vi "Main.vi"() -> ()   [LabVIEW 2017]
uses:
  TypeDefs/Listbox.ctl
  TypeDefs/Multicolumn.ctl
  TypeDefs/TabControl.ctl
  TypeDefs/Transparent String.ctl
  TypeDefs/DCP and LLDP Cluster.ctl
  TypeDefs/DCP ARRAY.ctl
  TypeDefs/Profinet Ident.ctl
  TypeDefs/LLDP ARRAY.ctl
  TypeDefs/LLDP.ctl
  Lib/WinPcap/lvwpcap.lvlib
panel:
  out "Program State":T1
  in  "Configuration Tab":bool
  in  "Scan Tab":bool
  in  "List of accessible devices:":T2
  in  "Tab Control":T3
  in  "Cancel Scan":bool
  in  "Network Adapters":T4
  in  "Scan Button":bool
  in  "Input parameter 3":string
  in  "Input parameter 2":string
  in  "Cancel Set":bool
  in  "Flash LED":bool
  in  "Set Button":bool
  in  "Input parameter 1":string
  in  "Choose Mode":T4
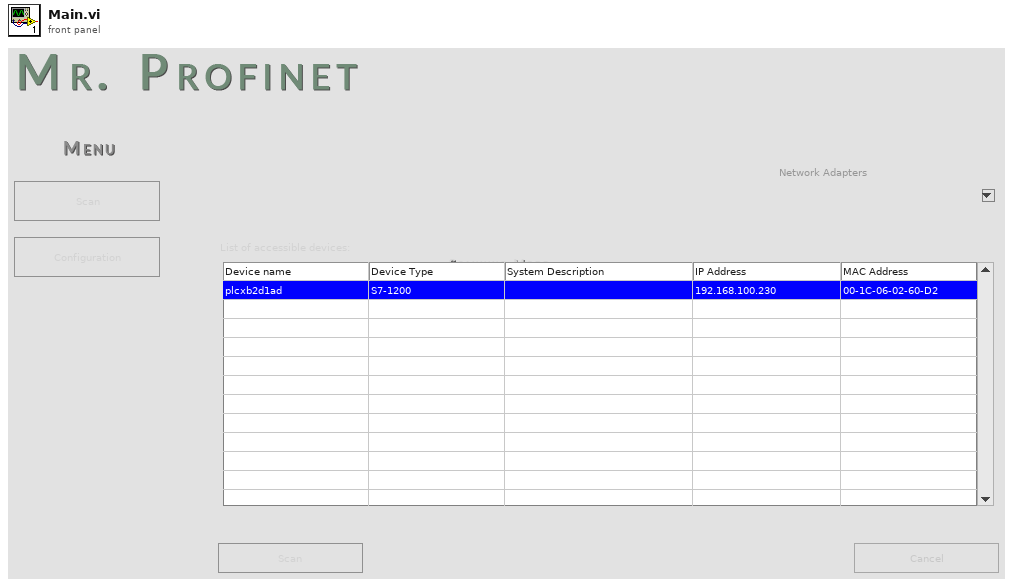
[diagram p1: front panel]
types:
  T1 = typedef "Transparent String.ctl" = string
  T2 = typedef "Multicolumn.ctl" = i32
  T3 = typedef "TabControl.ctl" = enum32{"Scan", "Configuration"}
  T4 = typedef "Listbox.ctl" = string
  T5 = enum32{"invalid app kind", "Development System", "Run Time System", "Student Edition", "Embedded LabVIEW", "Evaluation", "Custom"}
  T6 = enum8{"Enabled", "Disabled", "Disabled and Grayed Out"}
  T7 = enum32{"Invalid", "Standard", "Closed", "Hidden", "Minimized", "Maximized"}
  T8 = typedef "DCP and LLDP Cluster.ctl" = cluster{"DCP":T9, "LLDP":T11}
  T9 = typedef "DCP ARRAY.ctl" = T10[]
  T10 = typedef "Profinet Ident.ctl" = cluster{"Device Vendor Value":string, "Name Of Station":string, "IP Address":string, "Subnet Mask":string, "Default Gateway":string, "MAC Address":string, "MAC Address HEX":string, "System Description ":string}
  T11 = typedef "LLDP ARRAY.ctl" = T12[]
  T12 = typedef "LLDP.ctl" = cluster{"Chasis Subtype":string, "Port Subtype":string, "Port Description":string, "System Name":string, "System Description":string, "IP Address":string, "MAC Address":string, "MAC Address HEX":string}
  T13 = cluster{"Core":cluster{"Current VI Reference":refnum<vi>, "Close Panel on Exit?":bool}, "Scanner Data":T8, "Accesible Devices":string[][], "Interfaces":string[], "Interface index":i32, "Pcap Reference":u32, "Send parameters":cluster{"MAC Address":string, "Mode":string, "Parameter 1":string, "Parameter 2":string, "Parameter 3":string}}
  T14 = cluster{"MAC Address":string, "Mode":string, "Parameter 1":string, "Parameter 2":string, "Parameter 3":string}
  T15 = cluster{"Current VI Reference":refnum<vi>, "Close Panel on Exit?":bool}
  T16 = typedef "Control majster 5.ctl" = string
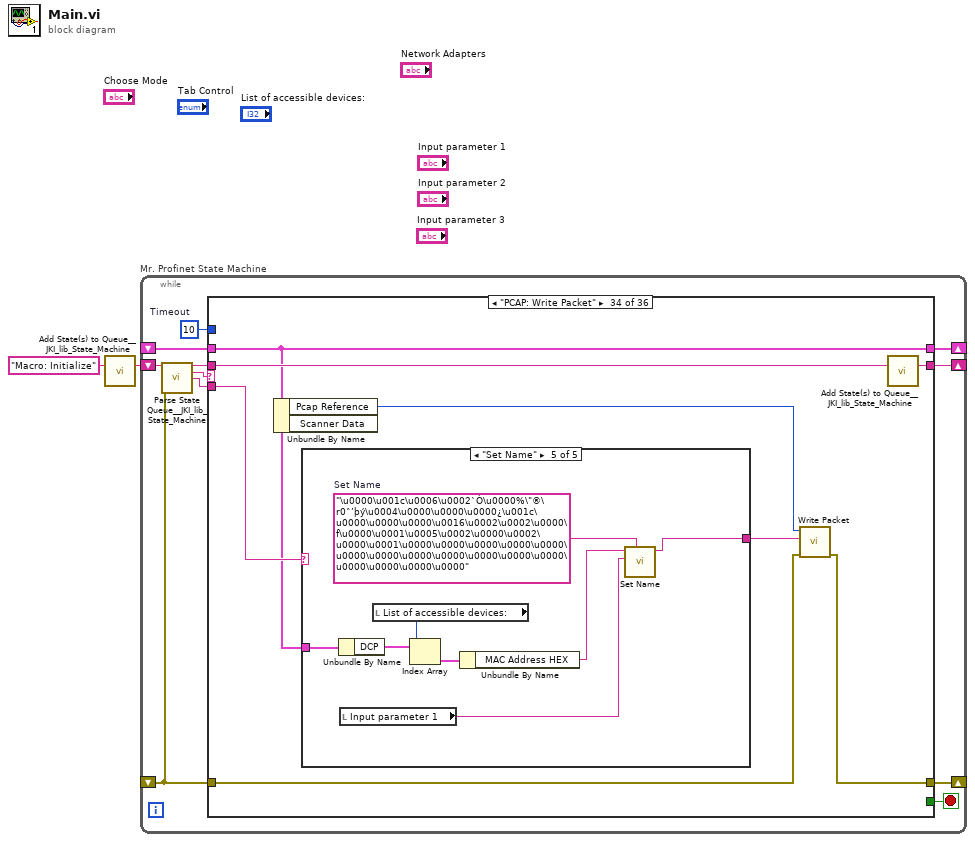
[diagram p0: block diagram]
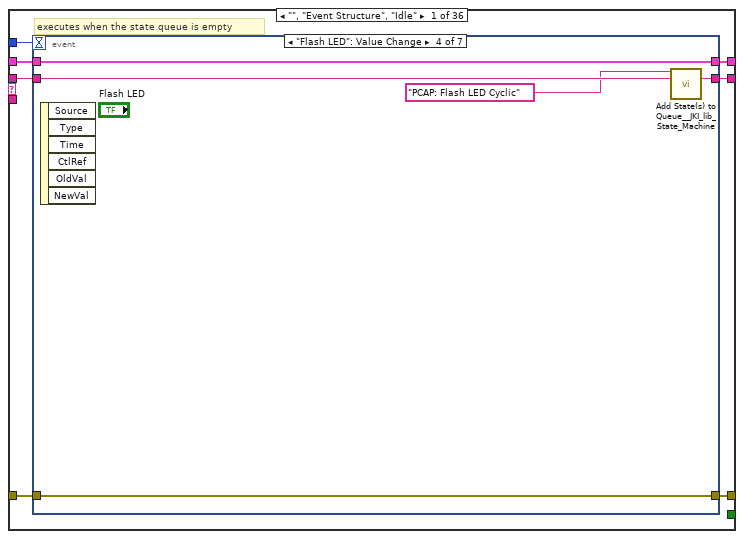
[diagram p2: hidden frame]
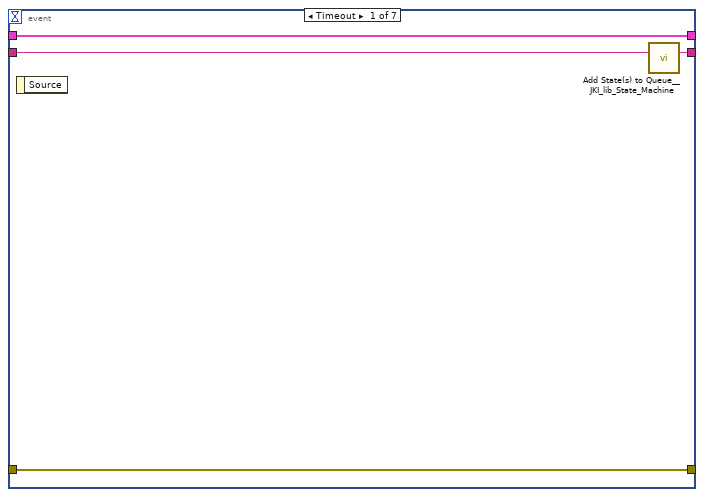
[diagram p3: hidden frame]
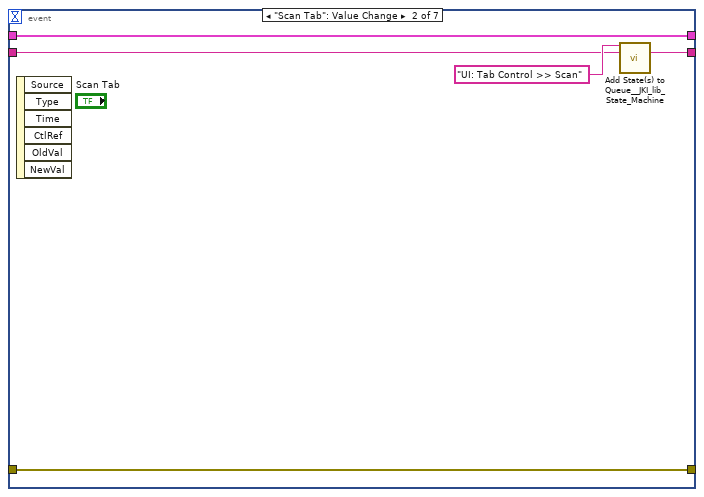
[diagram p4: hidden frame]
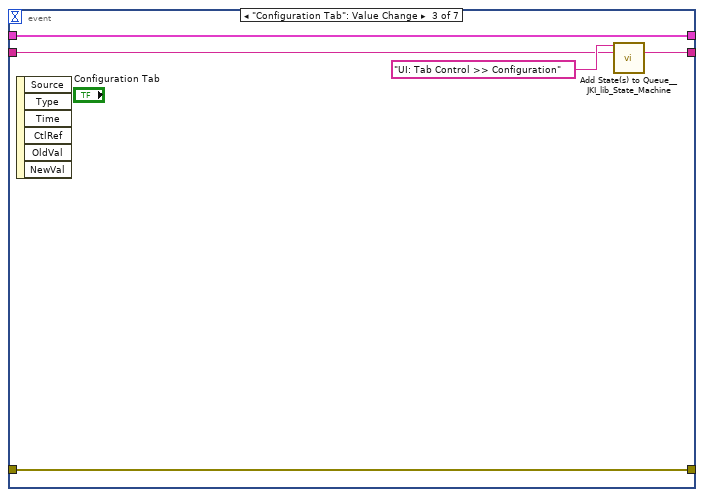
[diagram p5: hidden frame]
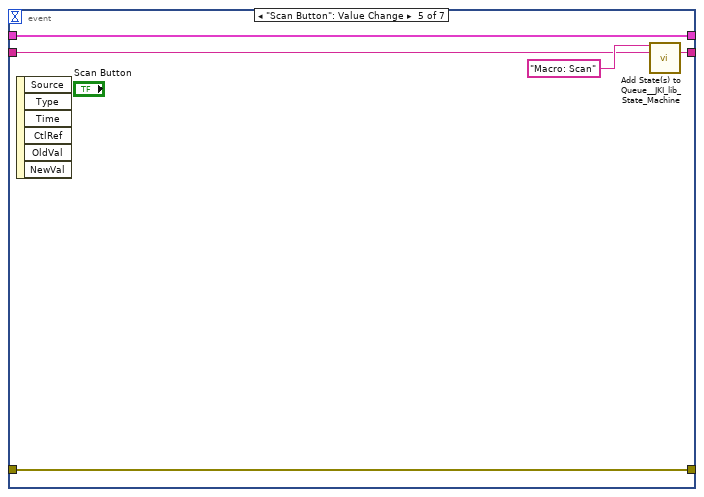
[diagram p6: hidden frame]
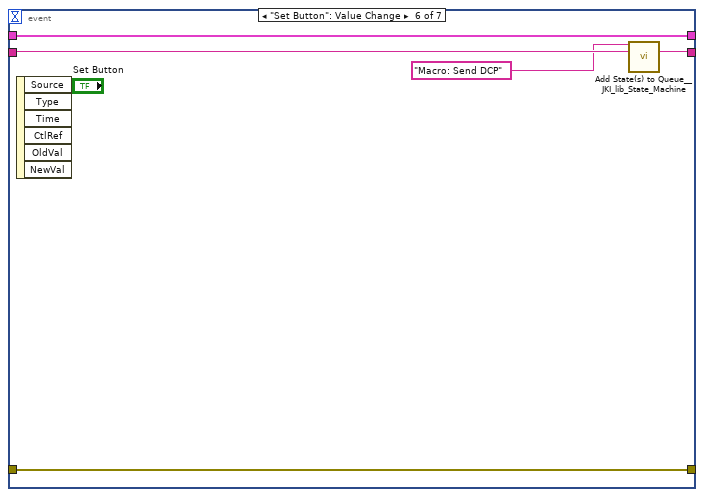
[diagram p7: hidden frame]
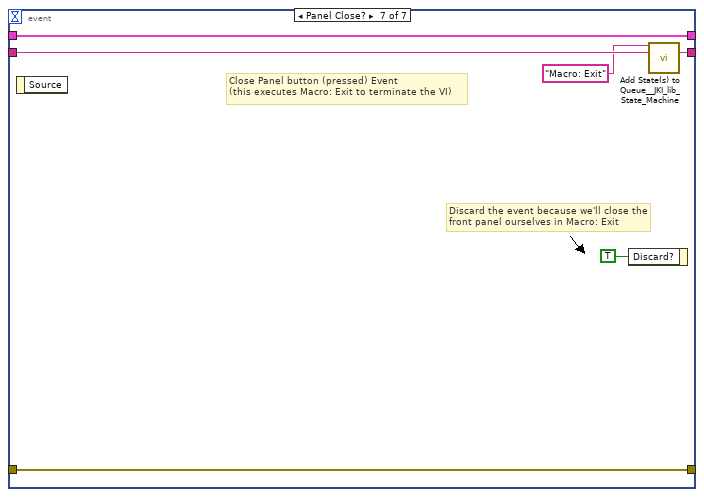
[diagram p8: hidden frame]
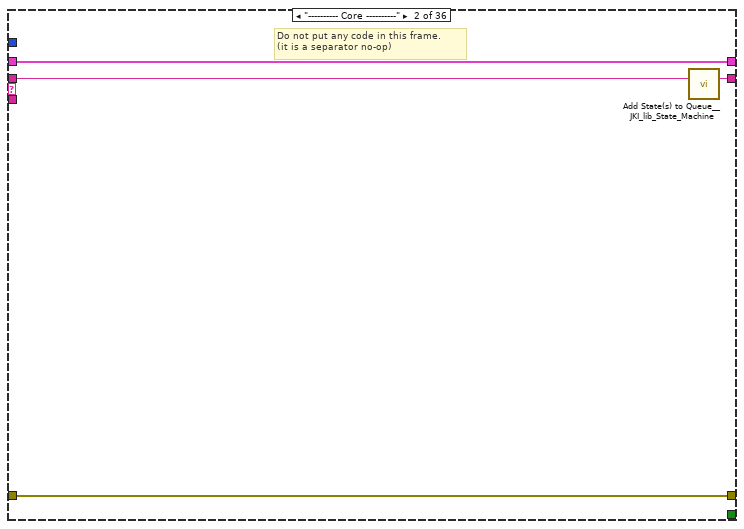
[diagram p9: hidden frame]
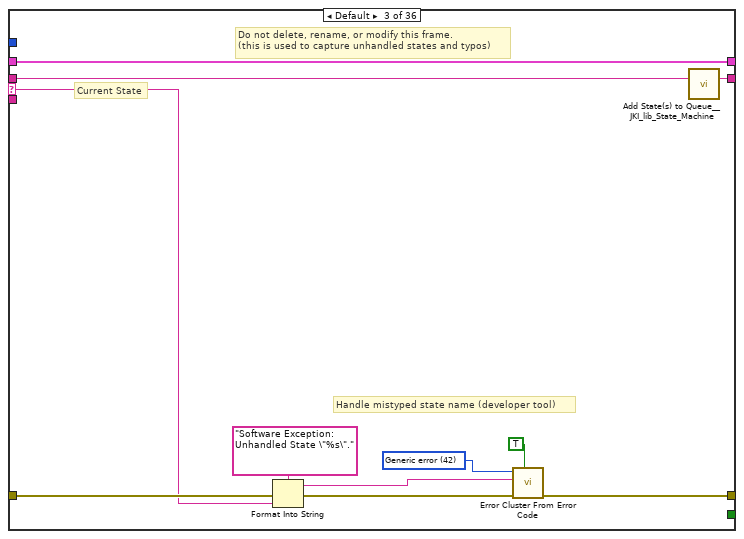
[diagram p10: hidden frame]
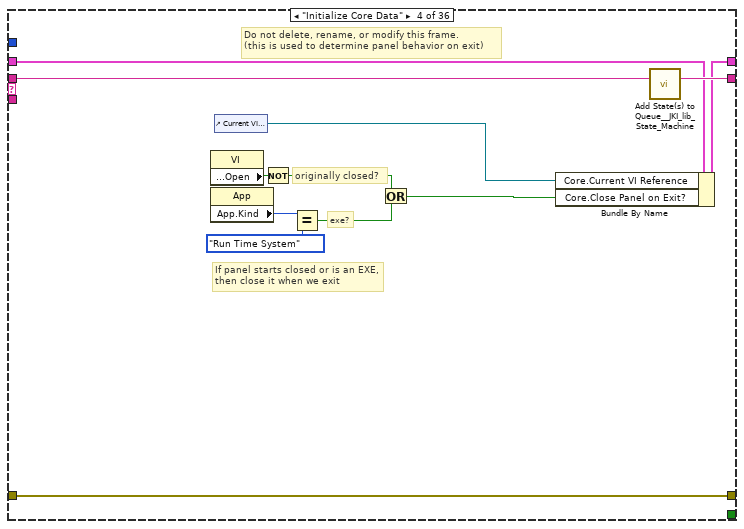
[diagram p11: hidden frame]
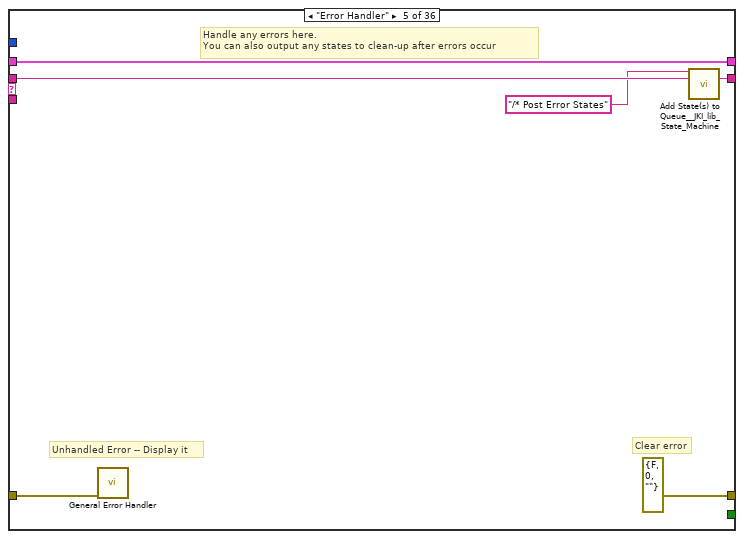
[diagram p12: hidden frame]
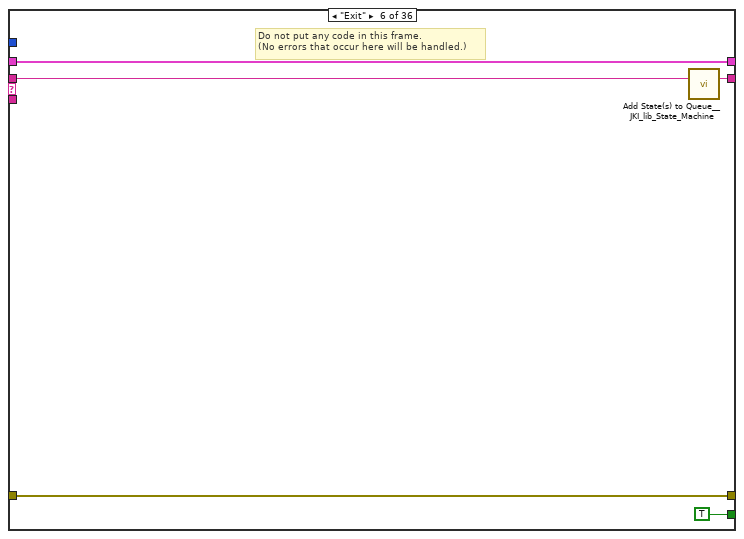
[diagram p13: hidden frame]
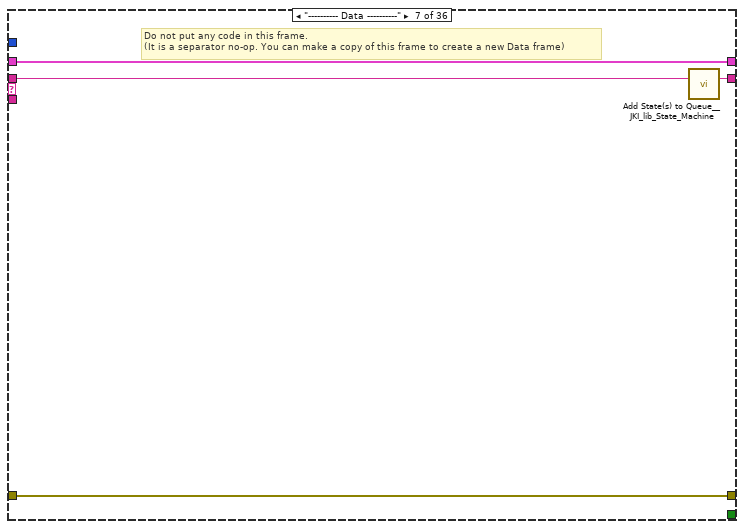
[diagram p14: hidden frame]
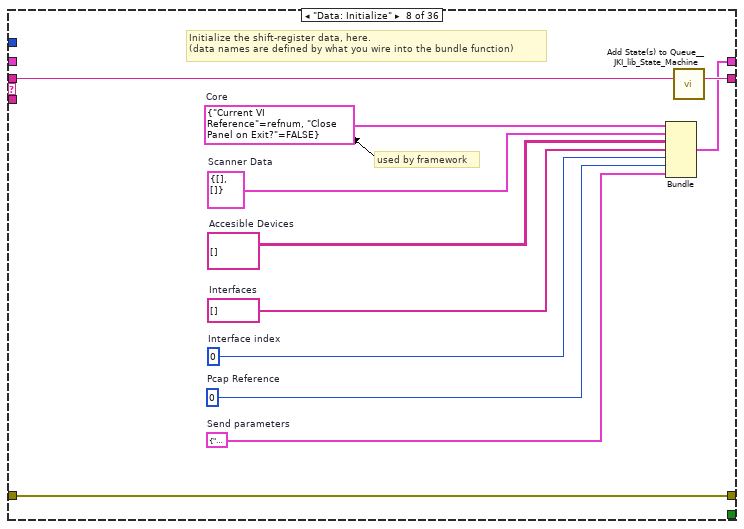
[diagram p15: hidden frame]
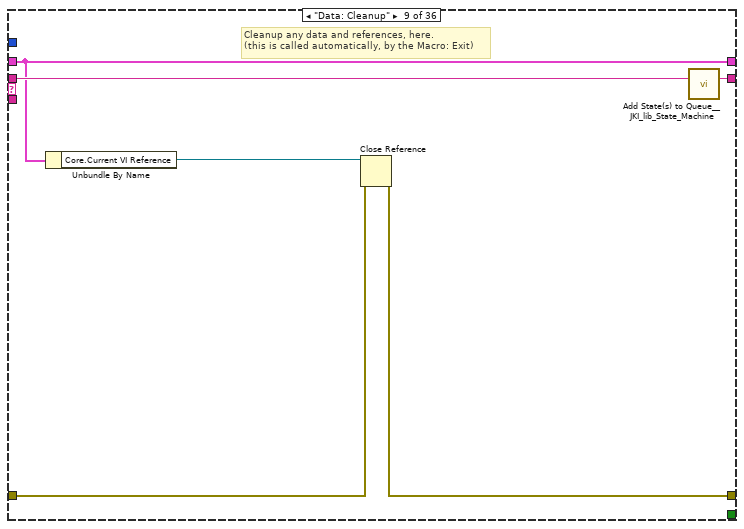
[diagram p16: hidden frame]
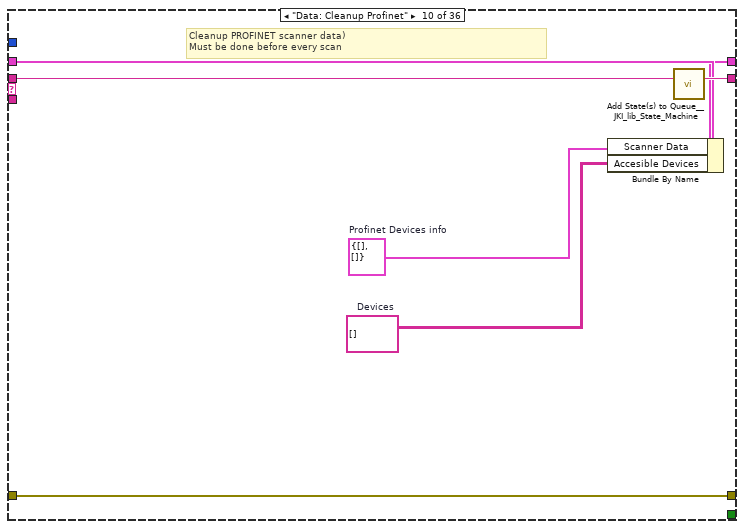
[diagram p17: hidden frame]
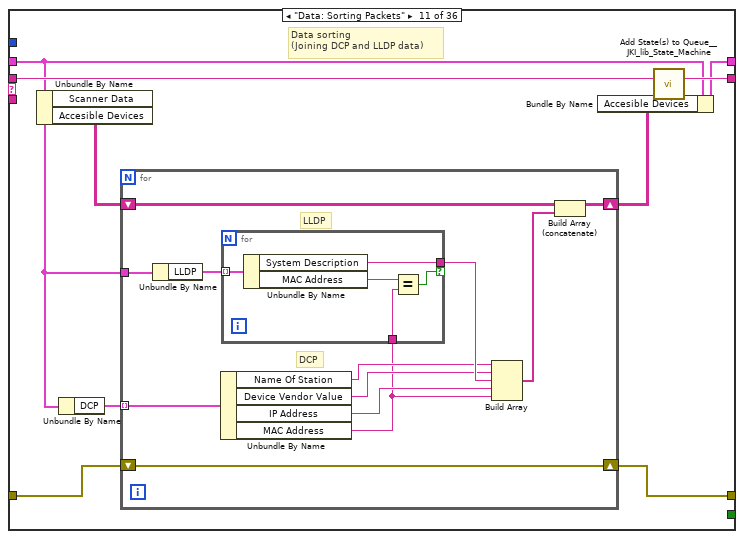
[diagram p18: hidden frame]
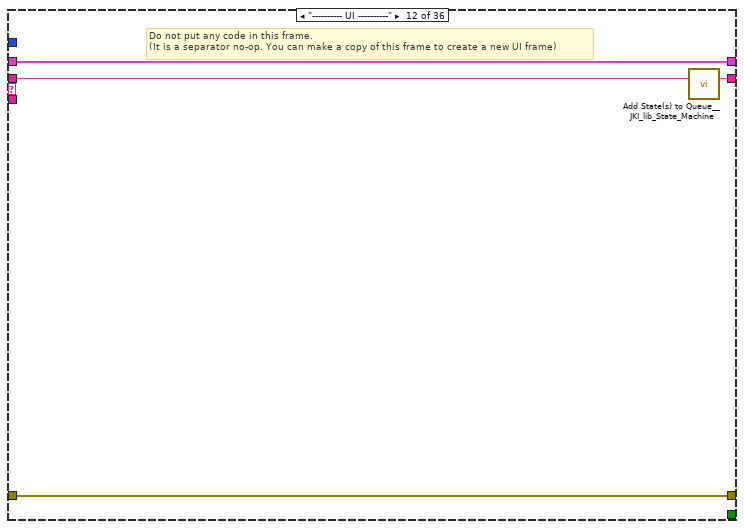
[diagram p19: hidden frame]
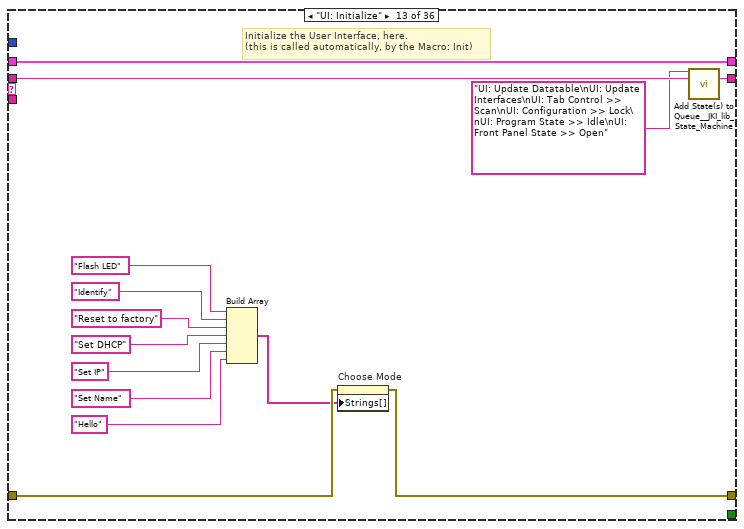
[diagram p20: hidden frame]
diagram:
  n1 = call <vilib>:"Add State(s) to Queue__JKI_lib_State_Machine.vi"("State(s) in (\"\")"="Macro: Initialize") -> ("States Out"=w2:string)  [unwired: 14 in]
  n2 = while "Mr. Profinet State Machine" {
    shift-right: [w6] -> _
    shift-left: _ -> [w5]
    shift-right: [w9] -> _
    shift-left: _ -> [w3]
    shift-right: [w8] -> _
    shift-left: w2 -> [w10]
    stop <- w7 stop-if-true
    w4 = 10  # Timeout
    n3 = call <vilib>:"Parse State Queue__JKI_lib_State_Machine.vi"("State Queue"=w10, "Error In (no error)"=w3) -> ("Remaining States"=w12:string, "Current State"=w13:string, "Arguments"=w11:string)  [unwired: 11 in]
    n4 = case shown="\"PCAP: Write Packet\"" w13 {
      selector: w13 -> [_ _ w60 _ _ _ _ _ _ _ _ _ _ _ _ _ _ _ _ _ _ _ _ _ _ _ _ _ _ _ _ _ _ _ _ _]
      tunnel: w12 -> [w20 w59 w64 w82 w88 w93 w97 w108 w114 w121 w131 w152 w166 w172 w178 w184 w194 w212 w230 w242 w252 w263 w289 w294 w299 w304 w312 w317 w327 w331 w345 w359 w366 w379 w425 w443]
      tunnel: w11 -> [_ _ _ _ _ _ _ _ _ _ _ _ _ _ _ w179 w189 w207 w225 w237 w247 w257 _ _ _ _ _ _ _ _ _ _ _ w373 _ _]
      tunnel: w5 -> [w18 w56 w62 w73 w85 w91 w94 _ w109 w118 w128 w149 w164 w170 w173 w182 w192 w210 w228 w240 w250 w259 w286 w291 w296 w301 w310 w314 w324 w328 w334 w352 w364 w377 w421 w438]
      tunnel: [w17 w57 w66 w79 errorcluster {"status"=FALSE, "code"=0, "source"=""} ("error out") w90 w95 w105 w110 w119 w126 w150 w161 w167 w174 w180 w190 w208 w226 w238 w248 w260 w287 w292 w297 w302 w308 w315 w325 w329 w336 w355 w362 w376 w418 w439] -> w9
      tunnel: w3 -> [w16 w57 w65 w79 w84 w90 w95 w105 w111 w119 w129 w150 w162 w168 w175 w181 w191 w209 w227 w239 w249 w261 w287 w292 w297 w302 w309 w315 w325 w329 w343 w356 w363 w375 w423 w441]
      tunnel: [w19 w58 w63 w81 w87 w92 w96 w107 w113 w120 w130 w151 w165 w171 w177 w183 w193 w211 w229 w241 w251 w262 w288 w293 w298 w303 w311 w316 w326 w330 w344 w358 w365 w378 w424 w442] -> w8
      tunnel: [_ _ _ _ _ TRUE _ _ _ _ _ _ _ _ _ _ _ _ _ _ _ _ _ _ _ _ _ _ _ _ _ _ _ _ _ _] -> w7
      tunnel: [w15 w56 w62 w80 w85 w91 w94 w106 w109 w116 w127 w149 w164 w170 w173 w182 w192 w210 w228 w240 w250 w259 w286 w291 w296 w301 w310 w314 w324 w328 w333 w351 w364 w377 w420 w438] -> w6
      tunnel: w4 -> [w14 _ _ _ _ _ _ _ _ _ _ _ _ _ _ _ _ _ _ _ _ _ _ _ _ _ _ _ _ _ _ _ _ _ _ _]
      frame "", "Event Structure", "Idle" {
        # "executes when the state queue is empty"
        n5 = event shown="[3] \"Flash LED\": Value Change" {
          selector: _ -> [_ _ _ _ _ _ _]
          dyn-events: _ -> [_ _ _ _ _ _ _]
          timeout: w14 -> [_ _ _ _ _ _ _]
          tunnel: w20 -> [w24 w25 w31 w37 w42 w47 w55]
          tunnel: [w23 w26 w32 w38 w43 w48 w54] -> w19
          tunnel: w18 -> [w21 w29 w34 w39 w41 w49 w52]
          tunnel: [w22 w28 w30 w36 w40 w45 w53] -> w17
          tunnel: w16 -> [w22 w28 w30 w36 w40 w45 w53]
          tunnel: [w21 w29 w34 w39 w41 w49 w52] -> w15
          event Timeout {
            n6 = event-data() -> ()  [unwired: 1 in, 1 out]
            n7 = call <vilib>:"Add State(s) to Queue__JKI_lib_State_Machine.vi"("State(s) in (\"\")"=w24) -> ("States Out"=w23:string)  [unwired: 14 in]
          }
          event "Scan Tab": Value Change {
            n8 = event-data() -> ()  [unwired: 1 in, 6 out]
            n9 = call <vilib>:"Add State(s) to Queue__JKI_lib_State_Machine.vi"("State(s) in Front (\"\")"="UI: Tab Control >> Scan", "State(s) in (\"\")"=w25) -> ("States Out"=w26:string)  [unwired: 13 in]
          }
          event "Configuration Tab": Value Change {
            n10 = event-data() -> ()  [unwired: 1 in, 6 out]
            n11 = call <vilib>:"Add State(s) to Queue__JKI_lib_State_Machine.vi"("State(s) in Front (\"\")"="UI: Tab Control >> Configuration", "State(s) in (\"\")"=w31) -> ("States Out"=w32:string)  [unwired: 13 in]
          }
          event "Flash LED": Value Change {
            n12 = event-data() -> ()  [unwired: 1 in, 6 out]
            n13 = call <vilib>:"Add State(s) to Queue__JKI_lib_State_Machine.vi"("State(s) in Front (\"\")"="PCAP: Flash LED Cyclic" ("State(s) in Front (\"\")"), "State(s) in (\"\")"=w37) -> ("States Out"=w38:string)  [unwired: 13 in]
          }
          event "Scan Button": Value Change {
            n14 = event-data() -> ()  [unwired: 1 in, 6 out]
            n15 = call <vilib>:"Add State(s) to Queue__JKI_lib_State_Machine.vi"("State(s) in Front (\"\")"="Macro: Scan", "State(s) in (\"\")"=w42) -> ("States Out"=w43:string)  [unwired: 13 in]
          }
          event "Set Button": Value Change {
            n16 = event-data() -> ()  [unwired: 1 in, 6 out]
            n17 = call <vilib>:"Add State(s) to Queue__JKI_lib_State_Machine.vi"("State(s) in Front (\"\")"="Macro: Send DCP", "State(s) in (\"\")"=w47) -> ("States Out"=w48:string)  [unwired: 13 in]
          }
          event Panel Close? {
            # "Discard the event because we'll close the front panel ourselves in Macro: Exit"
            # "Close Panel button (pressed) Event\n(this executes Macro: Exit to terminate the VI)"
            n18 = event-data() -> ()  [unwired: 1 in, 1 out]
            n19 = event-data("Discard?"=TRUE) -> ()  [unwired: 1 in, 1 out]
            n20 = call <vilib>:"Add State(s) to Queue__JKI_lib_State_Machine.vi"("State(s) in Front (\"\")"="Macro: Exit", "State(s) in (\"\")"=w55) -> ("States Out"=w54:string)  [unwired: 13 in]
          }
        }
      }
      frame "---------- Core ----------" {
        # "Do not put any code in this frame.\n(it is a separator no-op)"
        n21 = call <vilib>:"Add State(s) to Queue__JKI_lib_State_Machine.vi"("State(s) in (\"\")"=w59) -> ("States Out"=w58:string)  [unwired: 14 in]
      }
      frame Default {
        w69 = 42 items=["No error", "Argument error", "Memory is full", "Out of zone", "End of file", "File already open", "Generic file I/O error", "File not found", "File permission error", "Disk is full", "Duplicate path", "Too many files open", "System feature not enabled", "Resource file not found", "Cannot add resource", "Resource not found", "Image not found", "Image memory error", "Pen does not exist", "Config type invalid", "Config token not found", "Config parse error", "Config memory error", "Bad external code format", "Bad external code offset", "External code not present", "Null window", "Destroy window error", "Null menu", "Print aborted", "Bad print record", "Print driver error", "Windows error during printing", "Memory error during printing", "Print dialog error", "Generic print error", "Invalid device refnum", "Device not found", "Device parameter error", "Device unit error", "Cannot open device", "Device call aborted", "Generic error", "Cancelled by user", "Object ID too low", "Object ID too high", "Object not in heap", "Unknown heap", "Unknown object (invalid DefProc)", "Unknown object (DefProc not in table)", "Message out of range", "Invalid (null) method", "Unknown message", "Manager call not supported", "Bad address", "Network operation in progress", "Network operation timed out", "Connection is busy", "Network attribute not supported", "Network error", "Address in use", "System out of memory", "Connection aborted", "Connection refused", "Not connected", "Already connected", "Connection closed", "Initialization error (interapplication manager)", "Bad occurrence", "Wait on unbound occurrence handler", "Occurrence queue overflow", "Datalog type conflict", "Unused", "Unrecognized type (interapplication manager)", "Memory corrupt", "Failed to make temporary DLL", "Old CIN version", "Drag socket not found", "Failed to load drop-object", "Failed to register OLE object", "Failed to release OLE object", "Format specifier type mismatch", "Unknown format specifier", "Too few format specifiers", "Too many format specifiers", "Scan failed", "Newer CIN version", "Error converting to variant", "Runtime menu error", "Password tampered", "Variant attribute not found", "Incompatible variant data type", "Event data is not available", "Event Store is not present", "Occurrence is not found", "Event Queue is not created", "Event info is not available", "Refnum passed is NULL", "Error retrieving Class GUID", "Error retrieving CoClass GUID", "Error retrieving TypeLib GUID.", "Bad built application magic bytes.", "Specific driver is different from the specific driver associated with the Logical Name.", "There is no session opened to the class driver.", "Max Error", "MAX - Error with config objects", "MAX - Error loading configuration", "MAX - Group not supported"]
        # "Current State"
        # "Do not delete, rename, or modify this frame.\n(this is used to capture unhandled states and typos)"
        # "Handle mistyped state name (developer tool)"
        n22 = Format Into String(format string="Software Exception: Unhandled State \"%s\"." ("message"), error in=w65, w60) -> (resulting string=w68:string, error out=w67:errorcluster)  [unwired: 1 in]
        n23 = call <vilib>:"Error Cluster From Error Code.vi"("show call chain? (False)"=TRUE, "error in (no error)"=w67, "error message (\"\")"=w68, "error code (0)"=w69) -> ("error out"=w66:errorcluster)  [unwired: 5 in]
        n24 = call <vilib>:"Add State(s) to Queue__JKI_lib_State_Machine.vi"("State(s) in (\"\")"=w64) -> ("States Out"=w63:string)  [unwired: 14 in]
      }
      frame "Initialize Core Data" {
        # "Do not delete, rename, or modify this frame.\n(this is used to determine panel behavior on exit)"
        # "originally closed?"
        # "exe?"
        # "If panel starts closed or is an EXE, then close it when we exit"
        n25 = property class="VI"() -> ("Front Panel.Open"=w78:bool)  [unwired: 2 in, 2 out]
        n26 = property class="App"() -> ("App.Kind"=w77:T5)  [unwired: 2 in, 2 out]
        n27 = control-ref of="Current VI Reference"() -> (w71:refnum<vi>)
        n28 = Not(x=w78) -> (.not. x?=w75:bool)
        n29 = Equal?(x=w77, y=T5."Run Time System" ("Application:Kind")) -> (x = y?=w74:bool)
        n30 = Or(x=w75, y=w74) -> (x .or. y?=w72:bool)
        n31 = Bundle By Name(cluster=w73, "Core.Current VI Reference"=w71, "Core.Close Panel on Exit?"=w72) -> (w80:T13)
        n32 = call <vilib>:"Add State(s) to Queue__JKI_lib_State_Machine.vi"("State(s) in (\"\")"=w82) -> ("States Out"=w81:string)  [unwired: 14 in]
      }
      frame "Error Handler" {
        # "Unhandled Error -- Display it"
        # "Handle any errors here.\nYou can also output any states to clean-up after errors occur"
        # "Clear error"
        n33 = call <vilib>:"General Error Handler.vi"("error in (no error)"=w84) -> ()  [unwired: 10 in, 5 out]
        n34 = call <vilib>:"Add State(s) to Queue__JKI_lib_State_Machine.vi"("State(s) in Front (\"\")"="/* Post Error States", "State(s) in (\"\")"=w88) -> ("States Out"=w87:string)  [unwired: 13 in]
      }
      frame "Exit" {
        # "Do not put any code in this frame.\n(No errors that occur here will be handled.)"
        n35 = call <vilib>:"Add State(s) to Queue__JKI_lib_State_Machine.vi"("State(s) in (\"\")"=w93) -> ("States Out"=w92:string)  [unwired: 14 in]
      }
      frame "---------- Data ----------" {
        # "Do not put any code in this frame.\n(It is a separator no-op. You can make a copy of this frame to create a new Data frame)"
        n36 = call <vilib>:"Add State(s) to Queue__JKI_lib_State_Machine.vi"("State(s) in (\"\")"=w97) -> ("States Out"=w96:string)  [unwired: 14 in]
      }
      frame "Data: Initialize" {
        w98 = T14 {"MAC Address"="", "Mode"="", "Parameter 1"="", "Parameter 2"="", "Parameter 3"=""}  # Send parameters
        w99 = string[][] []  # Accesible Devices
        w104 = T8 {"DCP"=[], "LLDP"=[]}  # Scanner Data
        w102 = u32 0  # Pcap Reference
        w101 = 0  # Interface index
        w100 = string[] []  # Interfaces
        w103 = T15 {"Current VI Reference"=refnum, "Close Panel on Exit?"=FALSE}  # Core
        # "used by framework"
        # "Initialize the shift-register data, here.\n(data names are defined by what you wire into the bundle function)"
        n37 = Bundle("Core"=w103, "Scanner Data"=w104, "Accesible Devices"=w99, "Interfaces"=w100, "Interface index"=w101, "Pcap Reference"=w102, "Send parameters"=w98) -> (w106:T13)  [unwired: 1 in]
        n38 = call <vilib>:"Add State(s) to Queue__JKI_lib_State_Machine.vi"("State(s) in (\"\")"=w108) -> ("States Out"=w107:string)  [unwired: 14 in]
      }
      frame "Data: Cleanup" {
        # "Cleanup any data and references, here.\n(this is called automatically, by the Macro: Exit)"
        n39 = Unbundle By Name(w109) -> ("Core.Current VI Reference"=w112:refnum<vi>)
        n40 = Close Reference(reference=w112, error in (no error)=w111) -> (error out=w110:errorcluster)
        n41 = call <vilib>:"Add State(s) to Queue__JKI_lib_State_Machine.vi"("State(s) in (\"\")"=w114) -> ("States Out"=w113:string)  [unwired: 14 in]
      }
      frame "Data: Cleanup Profinet" {
        w115 = string[][] []  # Devices
        w117 = T8 {"DCP"=[], "LLDP"=[]}  # Profinet Devices info
        # "Cleanup PROFINET scanner data)\nMust be done before every scan"
        n42 = Bundle By Name(cluster=w118, "Scanner Data"=w117, "Accesible Devices"=w115) -> (w116:T13)
        n43 = call <vilib>:"Add State(s) to Queue__JKI_lib_State_Machine.vi"("State(s) in (\"\")"=w121) -> ("States Out"=w120:string)  [unwired: 14 in]
      }
      frame "Data: Sorting Packets" {
        # "Data sorting\n(Joining DCP and LLDP data)"
        n44 = Unbundle By Name(w128) -> ("Scanner Data"=w125:T8, "Accesible Devices"=w123:string[][])
        n45 = Unbundle By Name(w125) -> ("DCP"=w124:T9)
        n46 = for {
          shift-right: [w140] -> w126
          shift-left: w129 -> [w140]
          tunnel: w125 -> [w141]
          tunnel: w124 -> [w142] mode=indexing
          shift-right: [w139] -> w122
          shift-left: w123 -> [w138]
          # "DCP"
          # "LLDP"
          n47 = Unbundle By Name(w141) -> ("LLDP"=w143:T11)
          n48 = Unbundle By Name(w142) -> ("Name Of Station"=w136:string, "Device Vendor Value"=w135:string, "IP Address"=w134:string, "MAC Address"=w132:string)
          n49 = for {
            tunnel: w143 -> [w148] mode=indexing
            tunnel: [w146] -> w137 if=w145
            tunnel: w132 -> [w144]
            n50 = Unbundle By Name(w148) -> ("System Description"=w146:string, "MAC Address"=w147:string)
            n51 = Equal?(x=w147, y=w144) -> (x = y?=w145:bool)
          }
          n52 = Build Array(w136, w135, w137, w134, w132) -> (w133:string[])
          n53 = Build Array (concatenate)(w138, w133) -> (w139:string[][])
        }
        n54 = Bundle By Name(cluster=w128, "Accesible Devices"=w122) -> (w127:T13)
        n55 = call <vilib>:"Add State(s) to Queue__JKI_lib_State_Machine.vi"("State(s) in (\"\")"=w131) -> ("States Out"=w130:string)  [unwired: 14 in]
      }
      frame "---------- UI ----------" {
        # "Do not put any code in this frame.\n(It is a separator no-op. You can make a copy of this frame to create a new UI frame)"
        n56 = call <vilib>:"Add State(s) to Queue__JKI_lib_State_Machine.vi"("State(s) in (\"\")"=w152) -> ("States Out"=w151:string)  [unwired: 14 in]
      }
      frame "UI: Initialize" {
        # "Initialize the User Interface, here.\n(this is called automatically, by the Macro: Init)"
        n57 = Build Array("Flash LED", "Identify", "Reset to factory", "Set DHCP", "Set IP", "Set Name", "Hello") -> (w154:string[])
        n58 = property on="Choose Mode" class="CmbBox (strict)"(error in=w162, "Strings[]"=w154) -> (error out=w161:errorcluster)  [unwired: 1 in, 1 out]
        n59 = call <vilib>:"Add State(s) to Queue__JKI_lib_State_Machine.vi"("State(s) in Front (\"\")"="UI: Update Datatable\nUI: Update Interfaces\nUI: Tab Control >> Scan\nUI: Configuration >> Lock\nUI: Program State >> Idle\nUI: Front Panel State >> Open" ("State(s) in Front (\"\")"), "State(s) in (\"\")"=w166) -> ("States Out"=w165:string)  [unwired: 13 in]
      }
      frame "UI: Update Interfaces" {
        # "Initialize the User Interface, here.\n(this is called automatically, by the Macro: Init)"
        n60 = Unbundle By Name(w170) -> ("Interfaces"=w169:string[])
        n61 = property on="Network Adapters" class="CmbBox (strict)"(error in=w168, "Strings[]"=w169) -> (error out=w167:errorcluster)  [unwired: 1 in, 1 out]
        n62 = call <vilib>:"Add State(s) to Queue__JKI_lib_State_Machine.vi"("State(s) in (\"\")"=w172) -> ("States Out"=w171:string)  [unwired: 14 in]
      }
      frame "UI: Update Datatable" {
        # "Initialize the User Interface, here.\n(this is called automatically, by the Macro: Init)"
        n63 = Unbundle By Name(w173) -> ("Accesible Devices"=w176:string[][])
        n64 = property on="List of accessible devices:" class="MCListbox (strict)"(error in=w175, "ItemNames"=w176) -> (error out=w174:errorcluster)  [unwired: 1 in, 1 out]
        n65 = call <vilib>:"Add State(s) to Queue__JKI_lib_State_Machine.vi"("State(s) in (\"\")"=w178) -> ("States Out"=w177:string)  [unwired: 14 in]
      }
      frame "UI: Cursor Set" {
        # "Argument"
        # "Set and Unset Cursor Busy.\n(Usage: \"UI: Cursor Set >> Busy|Idle\")"
        n66 = case shown="\"Idle\", Default" w179 {
          tunnel: w181 -> [w186 w188]
          tunnel: [w185 w187] -> w180
          frame "Idle", Default {
            n67 = call <vilib>:"Unset Busy.vi"("error in (no error)"=w186) -> ("error out"=w185:errorcluster)  [unwired: 10 in]
          }
          frame "Busy" {
            n68 = call <vilib>:"Set Busy.vi"("error in (no error)"=w188) -> ("error out"=w187:errorcluster)  [unwired: 9 in, 1 out]
          }
        }
        n69 = call <vilib>:"Add State(s) to Queue__JKI_lib_State_Machine.vi"("State(s) in (\"\")"=w184) -> ("States Out"=w183:string)  [unwired: 14 in]
      }
      frame "UI: Scan State" {
        # "Set Scan State\n(Usage: \"UI: Scan State >> Busy|Idle\")"
        # "Argument"
        n70 = case shown="\"Busy\"" w189 {
          tunnel: w191 -> [w196 w202]
          tunnel: [w195 w201] -> w190
          frame "Idle", Default {
            n71 = property on="Cancel Scan" class="Bool (strict)"(error in=w196, "DisabledEnum"=T6."Disabled and Grayed Out" ("Disabled")) -> (error out=w200:errorcluster)  [unwired: 1 in, 1 out]
            n72 = property on="Scan Button" class="Bool (strict)"(error in=w200, "Value"=FALSE ("Set Tab"), "DisabledEnum"=T6."Enabled" ("Disabled")) -> (error out=w195:errorcluster)  [unwired: 1 in, 1 out]
          }
          frame "Busy" {
            n73 = property on="Scan Button" class="Bool (strict)"(error in=w202, "DisabledEnum"=T6."Disabled and Grayed Out" ("Disabled")) -> (error out=w206:errorcluster)  [unwired: 1 in, 1 out]
            n74 = property on="Cancel Scan" class="Bool (strict)"(error in=w206, "Value"=FALSE ("Set Tab"), "DisabledEnum"=T6."Enabled" ("Disabled")) -> (error out=w201:errorcluster)  [unwired: 1 in, 1 out]
          }
        }
        n75 = call <vilib>:"Add State(s) to Queue__JKI_lib_State_Machine.vi"("State(s) in (\"\")"=w194) -> ("States Out"=w193:string)  [unwired: 14 in]
      }
      frame "UI: Flash State" {
        # "Flash LED\n(Usage: \"UI: LED State >> Busy|Idle\")"
        # "Argument"
        n76 = case shown="\"Idle\", Default" w207 {
          tunnel: w209 -> [w214 w220]
          tunnel: [w213 w219] -> w208
          frame "Idle", Default {
            n77 = property on="Cancel Scan" class="Bool (strict)"(error in=w214, "DisabledEnum"=T6."Disabled and Grayed Out" ("Disabled")) -> (error out=w218:errorcluster)  [unwired: 1 in, 1 out]
            n78 = property on="Cancel Set" class="Bool (strict)"(error in=w218, "Value"=FALSE ("Set Tab"), "DisabledEnum"=T6."Enabled" ("Disabled")) -> (error out=w213:errorcluster)  [unwired: 1 in, 1 out]
          }
          frame "Busy" {
            n79 = property on="Set Button" class="Bool (strict)"(error in=w220, "DisabledEnum"=T6."Disabled and Grayed Out" ("Disabled")) -> (error out=w224:errorcluster)  [unwired: 1 in, 1 out]
            n80 = property on="Cancel Set" class="Bool (strict)"(error in=w224, "Value"=FALSE ("Set Tab"), "DisabledEnum"=T6."Enabled" ("Disabled")) -> (error out=w219:errorcluster)  [unwired: 1 in, 1 out]
          }
        }
        n81 = call <vilib>:"Add State(s) to Queue__JKI_lib_State_Machine.vi"("State(s) in (\"\")"=w212) -> ("States Out"=w211:string)  [unwired: 14 in]
      }
      frame "UI: Configuration" {
        # "Configuration Tab\n(Usage: \"UI: Configuration >> Lock|Unlock\")"
        # "Argument"
        n82 = case shown="\"Unlock\", Default" w225 {
          tunnel: w227 -> [w231 w235]
          tunnel: [w233 w234] -> w226
          frame "Unlock", Default {
            n83 = property on="Configuration Tab" class="Bool (strict)"(error in=w231, "DisabledEnum"=T6."Enabled" ("Disabled")) -> (error out=w233:errorcluster)  [unwired: 1 in, 1 out]
          }
          frame "Lock" {
            n84 = property on="Configuration Tab" class="Bool (strict)"(error in=w235, "DisabledEnum"=T6."Disabled and Grayed Out" ("Disabled")) -> (error out=w234:errorcluster)  [unwired: 1 in, 1 out]
          }
        }
        n85 = call <vilib>:"Add State(s) to Queue__JKI_lib_State_Machine.vi"("State(s) in (\"\")"=w230) -> ("States Out"=w229:string)  [unwired: 14 in]
      }
      frame "UI: Tab Control" {
        # "Configuration Tab\n(Usage: \"UI: Tab Control >> Tab|Tab\")"
        # "Argument"
        n86 = case shown="\"Scan\", Default" w237 {
          tunnel: w239 -> [w243 w246]
          tunnel: [w243 w246] -> w238
          frame "Scan", Default {
            n87 = local write "Tab Control"(TabControl."Scan" ("Tab Control")) -> ()
          }
          frame "Configuration" {
            n88 = local write "Tab Control"(TabControl."Configuration" ("Tab Control")) -> ()
          }
        }
        n89 = call <vilib>:"Add State(s) to Queue__JKI_lib_State_Machine.vi"("State(s) in (\"\")"=w242) -> ("States Out"=w241:string)  [unwired: 14 in]
      }
      frame "UI: Program State" {
        # "Argument"
        # "Set Program State\n(Usage: \"UI: Program State >> Busy|Idle\")"
        n90 = case shown="\"Idle\", Default" w247 {
          selector: w247 -> [w253 w255]
          tunnel: w249 -> [w254 w256]
          tunnel: [w254 w256] -> w248
          frame "Idle", Default {
            "Program State" <- w253
          }
          frame "Busy" {
            n91 = local write "Program State"(w255) -> ()
          }
        }
        n92 = call <vilib>:"Add State(s) to Queue__JKI_lib_State_Machine.vi"("State(s) in (\"\")"=w252) -> ("States Out"=w251:string)  [unwired: 14 in]
      }
      frame "UI: Front Panel State" {
        # "Argument"
        # "Set Front Panel Open or Closed\n(Usage: \"UI: Front Panel State >> Open|Close\")"
        n93 = Unbundle By Name(w259) -> ("Core.Current VI Reference"=w258:refnum<vi>)
        n94 = case shown="\"Open\", Default" w257 {
          tunnel: w261 -> [w267 w280]
          tunnel: [w269 w281] -> w260
          tunnel: w258 -> [w268 w278]
          frame "Open", Default {
            n95 = property class="VI"(reference=w268, error in=w267) -> (reference out=w265:refnum<vi>, error out=w266:errorcluster, "Front Panel.Open"=w264:bool)
            n96 = case shown="False" w264 {
              tunnel: [w272 w275] -> w269
              tunnel: w266 -> [w271 w275]
              tunnel: w265 -> [w270 _]
              frame False {
                n97 = invoke class="VI" method="FP.Open"(reference=w270, error in=w271, "Activate"=TRUE, "State"=T7."Standard") -> (error out=w272:errorcluster)  [unwired: 1 in, 4 out]
              }
              frame True {
              }
            }
          }
          frame "Close" {
            n98 = property class="VI"(reference=w278, error in=w280) -> (reference out=w277:refnum<vi>, error out=w279:errorcluster, "Front Panel.Open"=w276:bool)
            n99 = case shown="True" w276 {
              tunnel: [w282 w285] -> w281
              tunnel: w279 -> [w282 w284]
              tunnel: w277 -> [_ w283]
              frame False {
              }
              frame True {
                n100 = invoke class="VI" method="FP.Close"(reference=w283, error in=w284) -> (error out=w285:errorcluster)  [unwired: 1 in, 2 out]
              }
            }
          }
        }
        n101 = call <vilib>:"Add State(s) to Queue__JKI_lib_State_Machine.vi"("State(s) in (\"\")"=w263) -> ("States Out"=w262:string)  [unwired: 14 in]
      }
      frame "---------- Macro ----------" {
        # "Do not put any code in this frame.\n(It is a separator no-op. You can make a copy of this frame to create a new Macro frame)"
        n102 = call <vilib>:"Add State(s) to Queue__JKI_lib_State_Machine.vi"("State(s) in (\"\")"=w289) -> ("States Out"=w288:string)  [unwired: 14 in]
      }
      frame "Macro: Initialize" {
        # "Initialization Macro\n(This is called once, when the VI starts)"
        n103 = call <vilib>:"Add State(s) to Queue__JKI_lib_State_Machine.vi"("State(s) in Front (\"\")"="Data: Initialize\nInitialize Core Data\nPCAP: Init\nUI: Initialize\n", "State(s) in (\"\")"=w294) -> ("States Out"=w293:string)  [unwired: 13 in]
      }
      frame "Macro: Reinitialize" {
        # "Initialization Macro\n(This is called once, when the VI starts)"
        n104 = call <vilib>:"Add State(s) to Queue__JKI_lib_State_Machine.vi"("State(s) in Front (\"\")"="PCAP: Close Interface\nData: Initialize\nPCAP: Init\nUI: Initialize", "State(s) in (\"\")"=w299) -> ("States Out"=w298:string)  [unwired: 13 in]
      }
      frame "Macro: Flash LED" {
        w300 = "Data: Initialize\nInitialize Core Data\nPCAP: Init\nUI: Initialize\nUI: Front Panel State >> Open\nUI: Update Interfaces"  # Data: Initialize Initialize Core Data PCAP: Init UI: Initialize UI: Front Panel State >> Open UI: Update Interfaces
        # "Initialization Macro\n(This is called once, when the VI starts)"
        n105 = call <vilib>:"Add State(s) to Queue__JKI_lib_State_Machine.vi"("State(s) in Front (\"\")"=w300, "State(s) in (\"\")"=w304) -> ("States Out"=w303:string)  [unwired: 13 in]
      }
      frame "Macro: Send DCP" {
        # "Initialization Macro\n(This is called once, when the VI starts)"
        n106 = property on="Choose Mode" class="CmbBox (strict)"(error in=w309) -> (error out=w308:errorcluster, "Value"=w306:T16)  [unwired: 1 in, 1 out]
        n107 = Concatenate Strings("PCAP: Write Packet >> ", w306) -> (w305:string)
        n108 = call <vilib>:"Add State(s) to Queue__JKI_lib_State_Machine.vi"("State(s) in Front (\"\")"=w305, "State(s) in (\"\")"=w312) -> ("States Out"=w311:string)  [unwired: 13 in]
      }
      frame "Macro: Scan" {
        # "Initialization Macro\n(This is called once, when the VI starts)"
        n109 = call <vilib>:"Add State(s) to Queue__JKI_lib_State_Machine.vi"("State(s) in Front (\"\")"="UI: Program State >> Busy\nUI: Scan State >> Busy\nData: Cleanup Profinet \nPCAP: Open Interface\nPCAP: Write Packet >> Info Request\nPCAP: DCP Scanning\nData: Sorting Packets\nUI: Update Datatable\nUI: Scan State >> Idle\nUI: Configuration >> Unlock\nUI: Program State >> Idle\n\n", "State(s) in (\"\")"=w317) -> ("States Out"=w316:string)  [unwired: 13 in]
      }
      frame "Macro: Exit" {
        # "Exit Macro\n(This is called once, when the VI exits)"
        n110 = Unbundle By Name(w324) -> ("Core.Close Panel on Exit?"=w323:bool)
        n111 = Select(t="UI: Front Panel State >> Close", s=w323, f="") -> (s? t:f=w320:string)
        n112 = call <vilib>:"Add State(s) to Queue__JKI_lib_State_Machine.vi"("State(s) in (\"\")"=w320, "State(s) at Back (\"\")"="Data: Cleanup\nExit") -> ("States Out"=w318:string)  [unwired: 13 in]
        n113 = call <vilib>:"Add State(s) to Queue__JKI_lib_State_Machine.vi"("State(s) in Front (\"\")"=w318, "State(s) in (\"\")"=w327) -> ("States Out"=w326:string)  [unwired: 13 in]
      }
      frame "---------- WinPcap ----------" {
        # "Template Separator\n(You can make a copy of, or modify, this frame)"
        n114 = call <vilib>:"Add State(s) to Queue__JKI_lib_State_Machine.vi"("State(s) in (\"\")"=w331) -> ("States Out"=w330:string)  [unwired: 14 in]
      }
      frame "PCAP: Init" {
        n115 = call "Initialize.vi"("error in (no error)"=w343) -> ("error out"=w342:errorcluster)  [unwired: 10 in]
        n116 = call "Get Interface Count.vi"("error in (no error)"=w342) -> ("error out"=w341:errorcluster, "count"=w335:i32)  [unwired: 9 in]
        n117 = for {
          N: w335 -> [_]
          shift-right: [w347] -> w339
          shift-left: w341 -> [w348]
          tunnel: [w346] -> w340 mode=indexing
          i -> [w349]
          n118 = call "Get Interface.vi"("error in (no error)"=w348, "index"=w349) -> ("error out"=w347:errorcluster, "lvwpcap_interface_array"=w346:string[])  [unwired: 8 in]
        }
        n119 = Index Array(array=w340, index (col)=0 ("disabled index (col)")) -> (element=w338:string[])  [unwired: 1 in]
        n120 = call "Read Adapters Info Registry2.vi"("error in (no error)"=w339, "Array in"=w338, "Numeric"=w335) -> ("error out"=w336:errorcluster, "Array out"=w332:string[])  [unwired: 7 in]
        n121 = Bundle By Name(cluster=w334, "Interfaces"=w332) -> (w333:T13)
        n122 = call <vilib>:"Add State(s) to Queue__JKI_lib_State_Machine.vi"("State(s) in (\"\")"=w345) -> ("States Out"=w344:string)  [unwired: 14 in]
      }
      frame "PCAP: Open Interface" {
        w353 = 100  # read_timeout
        w354 = 1522  # capture_size
        # "Maximum ethernet frame size - 1522"
        n123 = Unbundle By Name(w352) -> ("Interface index"=w357:i32)
        n124 = call "Open Interface.vi"("read_timeout (1000)"=w353, "error in (no error)"=w356, "capture_size (65536)"=w354, "adapter (0)"=w357) -> ("error out"=w355:errorcluster, "pcap reference"=w350:u32)  [unwired: 6 in]
        n125 = Bundle By Name(cluster=w352, "Pcap Reference"=w350) -> (w351:T13)
        n126 = call <vilib>:"Add State(s) to Queue__JKI_lib_State_Machine.vi"("State(s) in (\"\")"=w359) -> ("States Out"=w358:string)  [unwired: 14 in]
      }
      frame "PCAP: Close Interface" {
        n127 = Unbundle By Name(w364) -> ("Pcap Reference"=w360:u32)
        n128 = Not A Number/Path/Refnum?(number/path/refnum=w360) -> (NaN/Path/Refnum?=w361:bool)
        n129 = case shown="False" w361 {
          tunnel: w360 -> [w369 _]
          tunnel: w363 -> [w368 w370]
          tunnel: [w367 w370] -> w362
          frame False {
            n130 = call "Close Interface.vi"("error in (no error)"=w368, "pcap reference"=w369) -> ("error out"=w367:errorcluster)  [unwired: 9 in]
          }
          frame True {
          }
        }
        n131 = call <vilib>:"Add State(s) to Queue__JKI_lib_State_Machine.vi"("State(s) in (\"\")"=w366) -> ("States Out"=w365:string)  [unwired: 14 in]
      }
      frame "PCAP: Write Packet" {
        n132 = Unbundle By Name(w377) -> ("Pcap Reference"=w374:u32, "Scanner Data"=w371:T8)
        n133 = case shown="\"Set Name\"" w373 {
          tunnel: [w384 "\u0001\u000eÏ\u0000\u0000\u0000\u0000%\"®\r0ˆ’þþ\u0005\u0000\u0000\u0000\u0000=\u0000À\u0000\u0004ÿÿ\u0000\u0000\u0000\u0000\u0000\u0000\u0000\u0000\u0000\u0000\u0000\u0000\u0000\u0000\u0000\u0000\u0000\u0000\u0000\u0000\u0000\u0000\u0000\u0000\u0000\u0000\u0000\u0000\u0000\u0000\u0000\u0000\u0000\u0000\u0000\u0000" w393 w401 w415] -> w372
          tunnel: w371 -> [w388 _ w396 w408 w414]
          frame "Flash LED" {
            w385 = "\u0000\u001c\u0006\u0002`Ò\u0000%\"®\r0ˆ’þý\u0004\u0000\u0000\u0000¸ç\u0000\u0000\u0000\b\u0005\u0003\u0000\u0004\u0000\u0000\u0001\u0000\u0000\u0000\u0000\u0000\u0000\u0000\u0000\u0000\u0000\u0000\u0000\u0000\u0000\u0000\u0000\u0000\u0000\u0000\u0000\u0000\u0000\u0000\u0000\u0000\u0000\u0000\u0000\u0000\u0000\u0000"  # Flash LED
            n134 = Unbundle By Name(w388) -> ("DCP"=w387:T9)
            n135 = local read "List of accessible devices:"() -> (w386:T2)
            n136 = Index Array(array=w387, index=w386) -> (element=w383:T10)
            n137 = Unbundle By Name(w383) -> ("MAC Address HEX"=w380:string)
            n138 = String Length(string=w380) -> (length=w382:i32)
            n139 = Replace Substring(2:w382, 3:0 ("offset (0)"), 4:w380, 5:w385) -> (1:w384:string)  [unwired: 1 out]
          }
          frame "Identify", Default {
          }
          frame "Reset to factory" {
            n140 = Unbundle By Name(w396) -> ("DCP"=w398:T9)
            n141 = local read "List of accessible devices:"() -> (w395:T2)
            n142 = Index Array(array=w398, index=w395) -> (element=w397:T10)
            n143 = Unbundle By Name(w397) -> ("MAC Address HEX"=w392:string)
            n144 = String Length(string=w392) -> (length=w391:i32)
            n145 = Replace Substring(2:w391, 3:0 ("offset (0)"), 4:w392, 5:"\u0000\u001c\u0006\u0002`Ò\u0000%\"®\r0ˆ’þý\u0004\u0000\u0000\u0000¿ö\u0000\u0000\u0000\u0006\u0005\u0005\u0000\u0002\u0000\u0000\u0000\u0000\u0000\u0000\u0000\u0000\u0000\u0000\u0000\u0000\u0000\u0000\u0000\u0000\u0000\u0000\u0000\u0000\u0000\u0000\u0000\u0000\u0000\u0000\u0000\u0000\u0000\u0000\u0000\u0000\u0000\u0000") -> (1:w393:string)  [unwired: 1 out]
          }
          frame "Set IP" {
            w404 = "\u0000\u001c\u0006\u0002`Ò\u0000%\"®\r0ˆ’þý\u0004\u0000\u0000\u0000¿z\u0000\u0000\u0000\u0012\u0001\u0002\u0000\u000e\u0000\u0001À¨dæÿÿÿ\u0000\u0000\u0000\u0000\u0000\u0000\u0000\u0000\u0000\u0000\u0000\u0000\u0000\u0000\u0000\u0000\u0000\u0000\u0000\u0000\u0000\u0000\u0000\u0000\u0000"  # Set IP Packet
            n146 = local read "List of accessible devices:"() -> (w406:T2)
            n147 = local read "Input parameter 1"() -> (w402:string)
            n148 = local read "Input parameter 2"() -> (w400:string)
            n149 = local read "Input parameter 3"() -> (w399:string)
            n150 = Unbundle By Name(w408) -> ("DCP"=w407:T9)
            n151 = Index Array(array=w407, index=w406) -> (element=w405:T10)
            n152 = Unbundle By Name(w405) -> ("MAC Address HEX"=w403:string)
            n153 = call "Set IP Address.vi"("Set IP Packet"=w404, "Input parameter 3"=w399, "Input parameter 2"=w400, "Input parameter 1"=w402, "MAC Address HEX"=w403) -> ("Output frame"=w401:string)  [unwired: 6 in]
          }
          frame "Set Name" {
            w416 = "\u0000\u001c\u0006\u0002`Ò\u0000%\"®\r0ˆ’þý\u0004\u0000\u0000\u0000¿\u001c\u0000\u0000\u0000\u0016\u0002\u0002\u0000\f\u0000\u0001\u0005\u0002\u0000\u0002\u0000\u0001\u0000\u0000\u0000\u0000\u0000\u0000\u0000\u0000\u0000\u0000\u0000\u0000\u0000\u0000\u0000\u0000"  # Set Name
            n154 = Unbundle By Name(w414) -> ("DCP"=w413:T9)
            n155 = local read "Input parameter 1"() -> (w409:string)
            n156 = local read "List of accessible devices:"() -> (w412:T2)
            n157 = Index Array(array=w413, index=w412) -> (element=w411:T10)
            n158 = Unbundle By Name(w411) -> ("MAC Address HEX"=w410:string)
            n159 = call "Set Name.vi"("Set IP Packet"=w416, "Input parameter 1"=w409, "MAC Address HEX"=w410) -> ("Output frame"=w415:string)  [unwired: 8 in]
          }
        }
        n160 = call "Write Packet.vi"("error in (no error)"=w375, "data to write"=w372, "pcap reference"=w374) -> ("error out"=w376:errorcluster)  [unwired: 7 in, 1 out]
        n161 = call <vilib>:"Add State(s) to Queue__JKI_lib_State_Machine.vi"("State(s) in (\"\")"=w379) -> ("States Out"=w378:string)  [unwired: 14 in]
      }
      frame "PCAP: DCP Scanning" {
        n162 = Unbundle By Name(w421) -> ("Pcap Reference"=w422:u32, "Scanner Data"=w417:T8)
        n163 = while {
          shift-right: [w430] -> w418
          shift-left: w423 -> [w436]
          tunnel: w422 -> [w435]
          shift-right: [w431] -> w419
          shift-left: w417 -> [w432]
          stop <- w428 stop-if-true
          # "Collected data >>"
          n164 = call "Read with parameters.vi"("error in (no error)"=w436, "pcap reference in"=w435) -> ("error out"=w433:errorcluster, "capture_data out"=w434:string)  [unwired: 7 in, 1 out]
          n165 = call "Elapsed Time"() -> ("Time has Elapsed"=w427:bool)  [unwired: 12 in, 7 out]
          n166 = call "Sorting Data new.vi"("Clusters in"=w432, "error in (no error)"=w433, "Data in"=w434) -> ("error out"=w430:errorcluster, "Clusters out"=w431:T8)  [unwired: 5 in]
          n167 = Unbundle By Name(w430) -> ("status"=w429:bool)
          n168 = Compound Arithmetic op=OR(w429, "Cancel Scan", w427) -> (w428:bool)
        }
        n169 = Bundle By Name(cluster=w421, "Scanner Data"=w419) -> (w420:T13)
        n170 = call <vilib>:"Add State(s) to Queue__JKI_lib_State_Machine.vi"("State(s) in (\"\")"=w425) -> ("States Out"=w424:string)  [unwired: 14 in]
      }
      frame "PCAP: Flash LED Cyclic" {
        n171 = Unbundle By Name(w438) -> ("Pcap Reference"=w440:u32, "Scanner Data"=w437:T8)
        n172 = while {
          shift-right: [w454] -> w439
          shift-left: w441 -> [w452]
          tunnel: w440 -> [w455]
          tunnel: w437 -> [w444]
          stop <- w458 stop-if-true
          n173 = Unbundle By Name(w444) -> ("DCP"=w450:T9)
          n174 = local read "List of accessible devices:"() -> (w449:T2)
          n175 = Index Array(array=w450, index=w449) -> (element=w448:T10)
          n176 = Unbundle By Name(w448) -> ("MAC Address HEX"=w447:string)
          n177 = call "Flash LED.vi"("MAC Address in Hex"=w447, "error in (no error)"=w452) -> ("Flash LED Frame"=w446:string, "error out"=w451:errorcluster)  [unwired: 5 in]
          n178 = call "Elapsed Time 2"() -> ("Time has Elapsed"=w457:bool)  [unwired: 12 in, 7 out]
          n179 = call "Write Packet.vi"("error in (no error)"=w451, "data to write"=w446, "pcap reference"=w455) -> ("error out"=w454:errorcluster)  [unwired: 7 in, 1 out]
          n180 = Unbundle By Name(w454) -> ("status"=w453:bool)
          n181 = Wait (ms)(milliseconds to wait=u32 500) -> ()  [unwired: 1 out]
          n182 = Compound Arithmetic op=OR(w453, "Cancel Set", w457) -> (w458:bool)
        }
        n183 = call <vilib>:"Add State(s) to Queue__JKI_lib_State_Machine.vi"("State(s) in (\"\")"=w443) -> ("States Out"=w442:string)  [unwired: 14 in]
      }
    }
  }
